vi "EnterComments.vi"() -> (1 "update?":bool)   [LabVIEW 2018]
panel:
  out "Other comments made so far:":string
  in  "stop":bool
  in  "Add":bool
  in  "Comment:":string
  # "PLEASE ENTER YOUR COMMENT:"
  # "(ESC)"
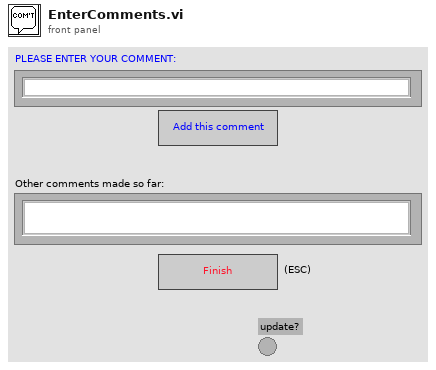
[diagram p1: front panel]
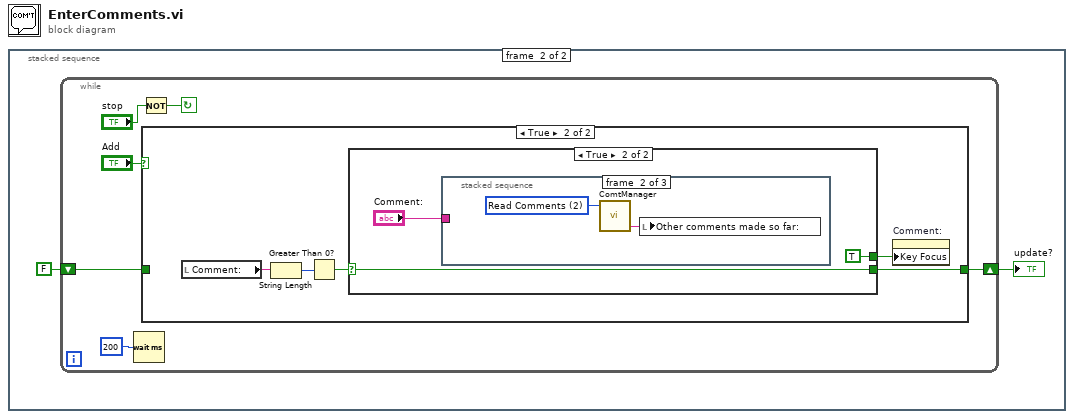
[diagram p0: block diagram]
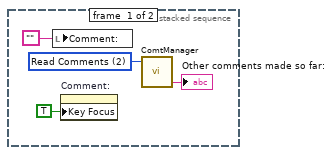
[diagram p2: hidden frame]
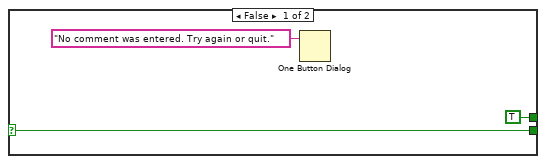
[diagram p4: hidden frame]
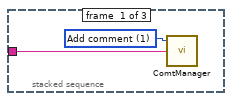
[diagram p5: hidden frame]
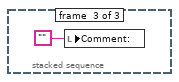
[diagram p6: hidden frame]
diagram:
  n1 = stacked-sequence {
    frame #0 {
      w2 = u16 2 items=["Initialise", "Add comment", "Read Comments"] ("Action")
      n2 = local write "Comment:"("") -> ()
      n3 = property on="Comment:" class="Str"("Key Focus"=TRUE) -> ()  [unwired: 2 in, 2 out]
      n4 = call "ComtManager.vi"("Action"=w2) -> ("Comment out"=→"Other comments made so far:":string)  [unwired: 2 in, 2 out]
    }
    frame #1 {
      n5 = while {
        shift-right: [w8] -> w6
        shift-left: FALSE -> [w7]
        stop <- w11 continue-if-true
        n6 = Wait (ms)(milliseconds to wait=u32 200) -> ()  [unwired: 1 out]
        n7 = Not(x="stop") -> (.not. x?=w11:bool)
        n8 = case shown="True" "Add" {
          tunnel: [w13 w18] -> w8
          tunnel: w7 -> [w13 _]
          frame False {
          }
          frame True {
            n9 = local read "Comment:"() -> (w17:string)
            n10 = String Length(string=w17) -> (length=w16:i32)
            n11 = Greater Than 0?(x=w16) -> (x > 0?=w15:bool)
            n12 = case shown="True" w15 {
              selector: w15 -> [w19 w22]
              tunnel: [w19 w22] -> w18
              tunnel: [TRUE ("Key Focus") TRUE ("Key Focus")] -> w14
              frame False {
                n13 = One Button Dialog(message="No comment was entered. Try again or quit.") -> ()  [unwired: 1 in, 1 out]
              }
              frame True {
                n14 = stacked-sequence {
                  tunnel: "Comment:" -> [w25 _ _]
                  frame #0 {
                    w26 = u16 1 items=["Initialise", "Add comment", "Read Comments"] ("Action")
                    n15 = call "ComtManager.vi"("Comment in"=w25, "Action"=w26) -> ()  [unwired: 1 in, 3 out]
                  }
                  frame #1 {
                    w28 = u16 2 items=["Initialise", "Add comment", "Read Comments"] ("Action")
                    n16 = call "ComtManager.vi"("Action"=w28) -> ("Comment out"=w27:string)  [unwired: 2 in, 2 out]
                    n17 = local write "Other comments made so far:"(w27) -> ()
                  }
                  frame #2 {
                    n18 = local write "Comment:"("") -> ()
                  }
                }
              }
            }
            n19 = property on="Comment:" class="Str"("Key Focus"=w14) -> ()  [unwired: 2 in, 2 out]
          }
        }
      }
      "update?" <- w6
    }
  }
